vi "QSPARK_laserStatusMonitor.vi"(11 "client handle":T1) -> (1 "laser on?":bool, 2 "remaining pulses":i32, 3 "client handle out":T1)   [LabVIEW 2024]
uses:
  <vilib>/httpClient/LabVIEWHTTPClient.lvlib
  <vilib>/httpClient/ClientHandle.ctl
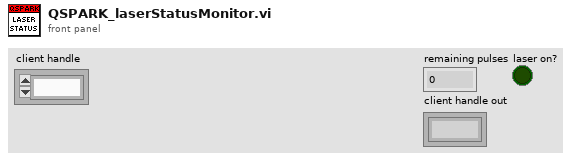
[diagram p1: front panel]
types:
  T1 = typedef "LabVIEWHTTPClient.lvlib/ClientHandle.ctl" = refnum<k1>
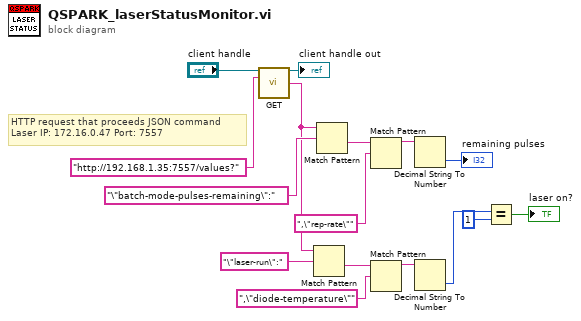
[diagram p0: block diagram]
diagram:
  # "HTTP request that proceeds JSON command\nLaser IP: 172.16.0.47 Port: 7557"
  n1 = call <vilib>:"GET.vi"("client handle"="client handle", "url"="http://192.168.1.35:7557/values?") -> ("client handle out"=→"client handle out":T1, "body"=w7:string)  [unwired: 10 in, 2 out]
  n2 = Match Pattern(string=w7, regular expression="\"laser-run\":") -> (after substring=w13:string)  [unwired: 1 in, 3 out]
  n3 = Match Pattern(string=w7, regular expression="\"batch-mode-pulses-remaining\":") -> (after substring=w10:string)  [unwired: 1 in, 3 out]
  n4 = Match Pattern(string=w10, regular expression=",\"rep-rate\"") -> (before substring=w8:string)  [unwired: 1 in, 3 out]
  n5 = Match Pattern(string=w13, regular expression=",\"diode-temperature\"") -> (before substring=w12:string)  [unwired: 1 in, 3 out]
  n6 = Decimal String To Number(string=w8) -> (number=→"remaining pulses":i32)  [unwired: 2 in, 1 out]
  n7 = Decimal String To Number(string=w12) -> (number=w6:i32)  [unwired: 2 in, 1 out]
  n8 = Equal?(x=w6, y=1) -> (x = y?=→"laser on?":bool)
